vi "DCON Action Engine.vi"(4 "Index\\Channel":i32, 5 "AO Value":dbl, 6 "Action":T4, 7 "DAQDevices":T3[](array[typedef]), 8 "error in (no error)":errorcluster, 9 "DO Value":bool, 10 "Device Name":T1, 11 "IO In":refnum<class "IO.lvclass">) -> (0 "error out":errorcluster, 1 "Status Out":T2, 2 "Channel Data":variant, 3 "IO Out":refnum<class "IO.lvclass">)   [LabVIEW 2022 SP3, in "IO.lvclass"]
uses:
  IO.lvclass
  Typedefs/DCON Action Engine-States.ctl
  Typedefs/DCON_DeviceConfig--Cluster.ctl
  Typedefs/DCON Private Data.ctl
  Typedefs/Device Names.ctl
  <vilib>/Instr/_visa.llb/VISA Flush IO Buffer Mask.ctl
  98b29336-fba3-426d-ab06-4e330d8353b0.vi
  <userlib>/_OpenG.lib/array/array.llb/Remove Duplicates from 1D Array (String)__ogtk.vi
  <userlib>/_OpenG.lib/array/array.llb/Delete Elements from 1D Array (U32)__ogtk.vi
  <vilib>/Instr/_visa.llb/VISA Configure Serial Port (Instr).vi
panel:
  out "read buffer 4":string
  out "read buffer 3":string
  out "read buffer 2":string
  out "read buffer":string
  out "output 1":i32
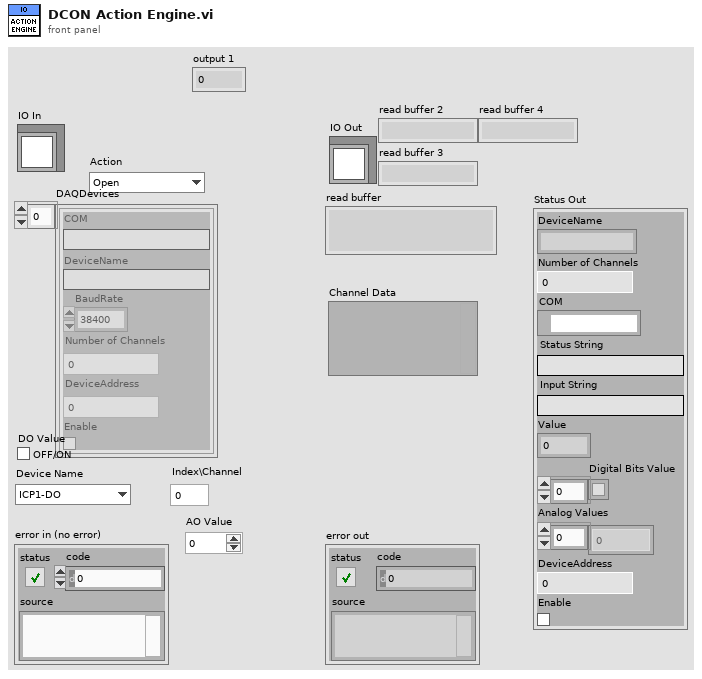
[diagram p1: front panel]
types:
  T1 = typedef "IO.lvclass/Device Names.ctl" = enum16{"ICP1-DO", "ICP2-DI", "ICP2-DO", "ICP1-AI", "ICP1-AO", "ICP2-AO"}
  T2 = typedef "IO.lvclass/DCON Private Data.ctl" = cluster{"DeviceName":string, "Number of Channels":i32, "COM":refnum<visa-resource-name>, "Status String":string, "Input String":string, "Value ":i32, "Digital Bits Value":bool[], "Analog Values":dbl[], "DeviceAddress":i32, "Enable":bool}
  T3 = typedef "IO.lvclass/DCON_DeviceConfig--Cluster.ctl" = cluster{"COM":string, "DeviceName":string, "BaudRate":u32, "Number of Channels":i32, "DeviceAddress":i32, "Enable":bool}
  T4 = typedef "DCON Action Engine-States.ctl" = enum16{"Open", "Close", "Set DO Value", "Get Digital Status", "Get Data", "Get AI Status", "Set AO Value", "Get AO Status"}
  T5 = typedef "VISA Flush IO Buffer Mask.ctl" = u16
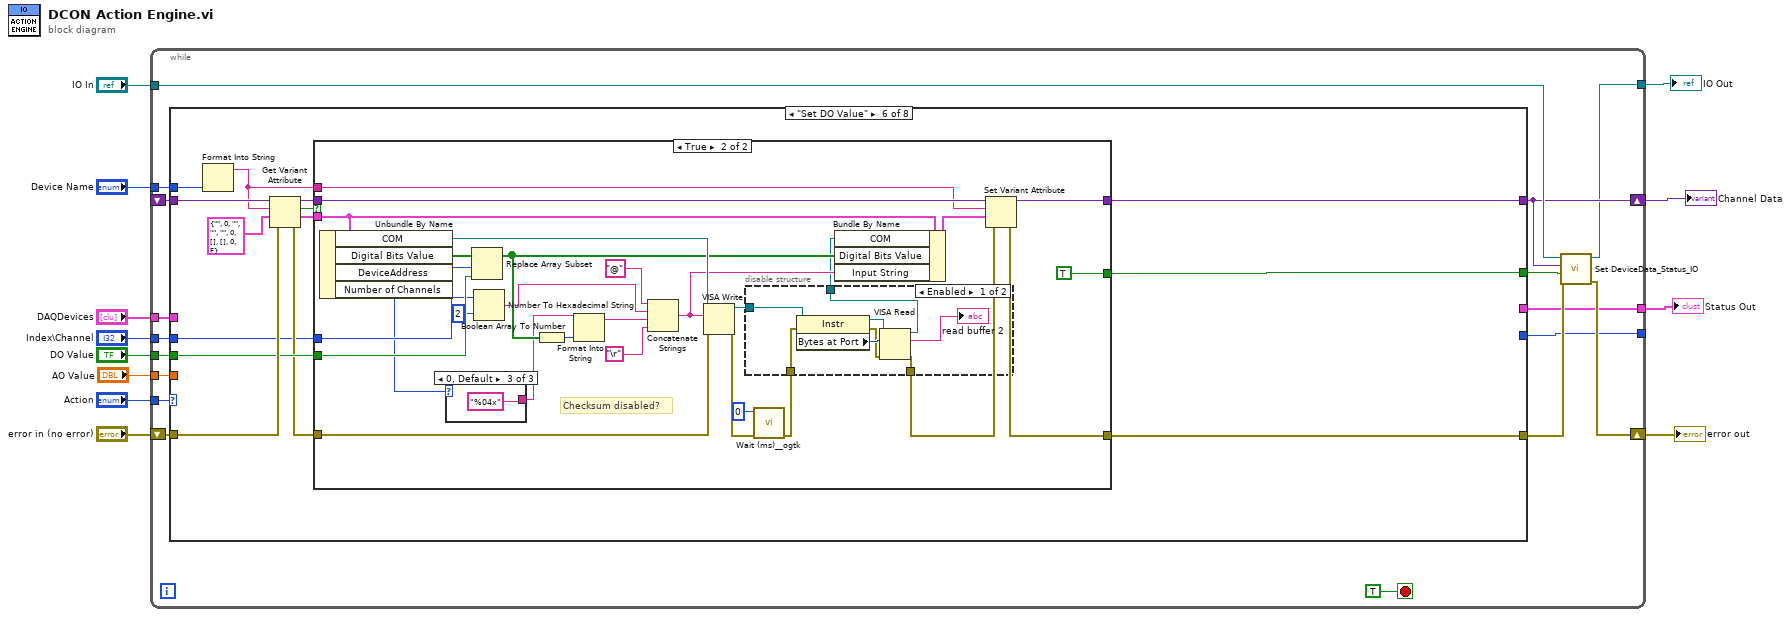
[diagram p0: block diagram]
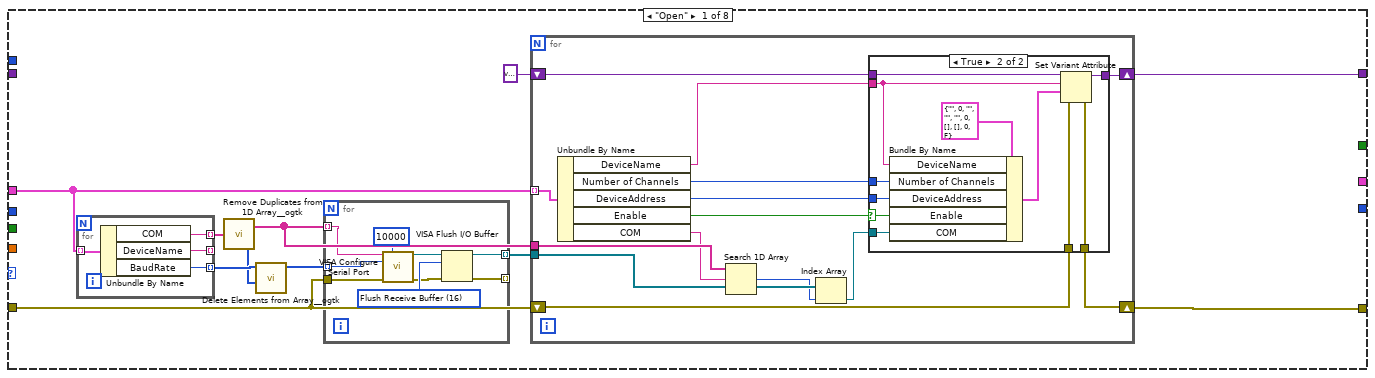
[diagram p2: hidden frame]
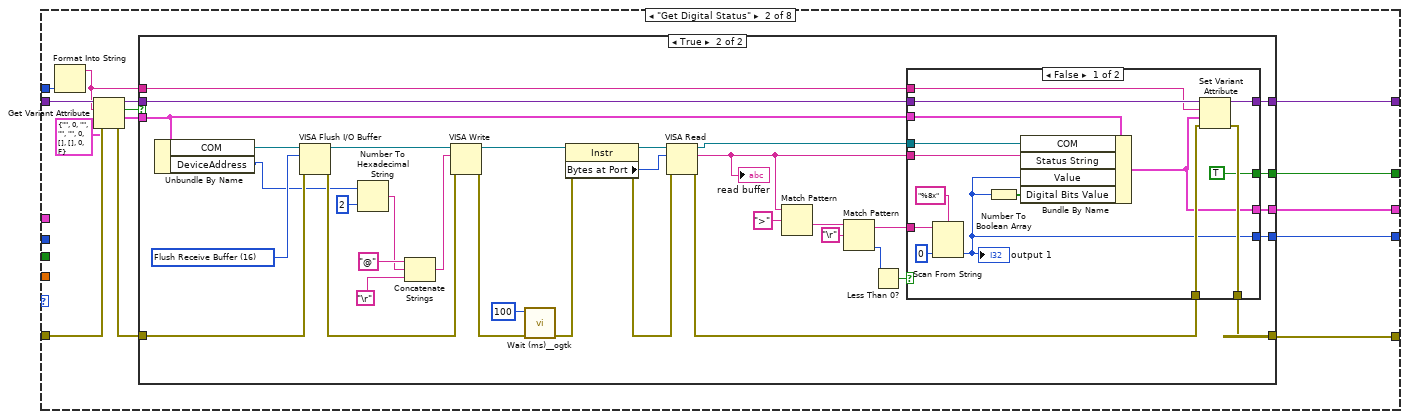
[diagram p4: hidden frame]
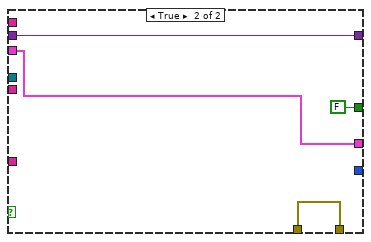
[diagram p6: hidden frame]
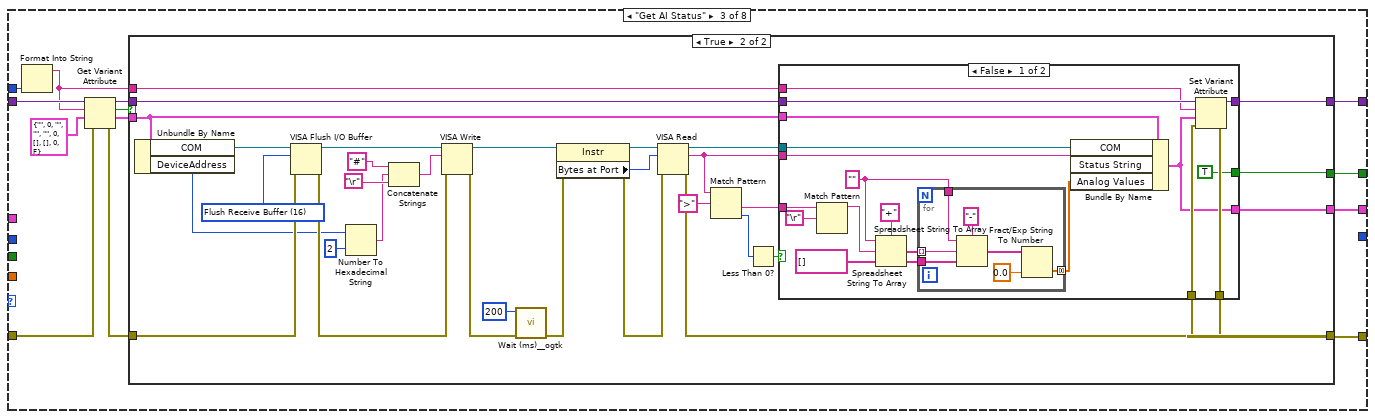
[diagram p7: hidden frame]
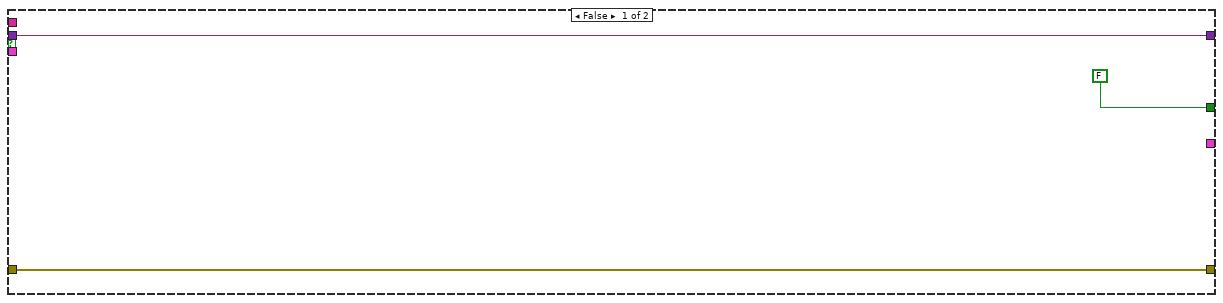
[diagram p8: hidden frame]
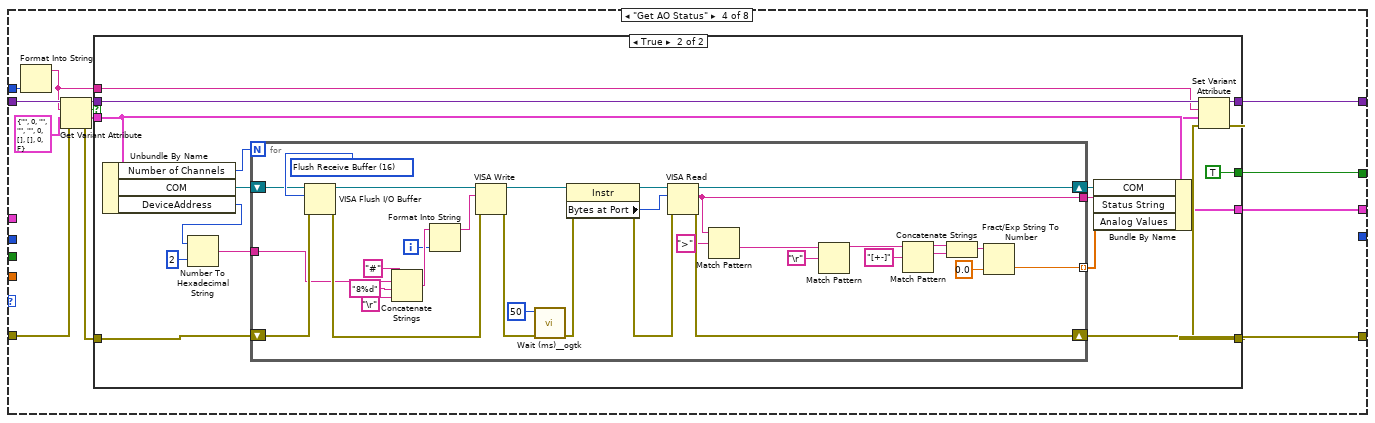
[diagram p10: hidden frame]
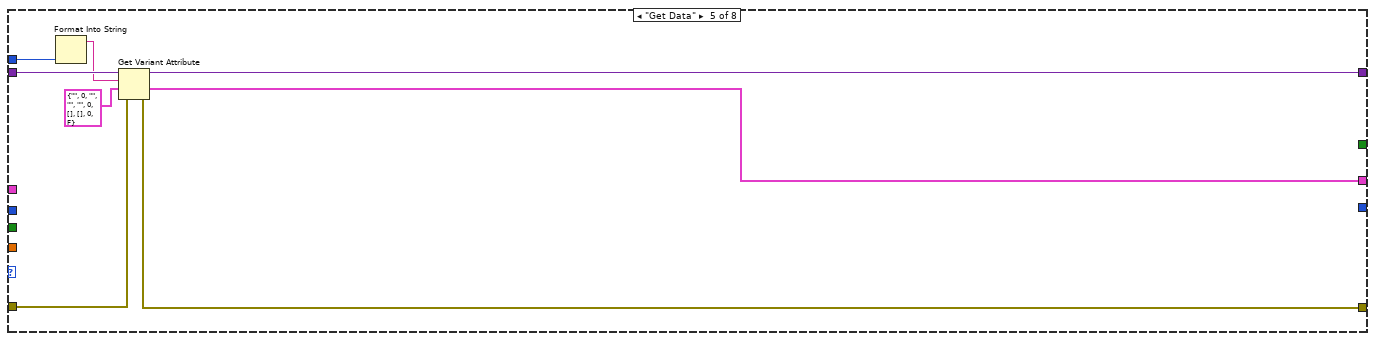
[diagram p12: hidden frame]
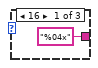
[diagram p14: hidden frame]
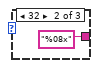
[diagram p15: hidden frame]
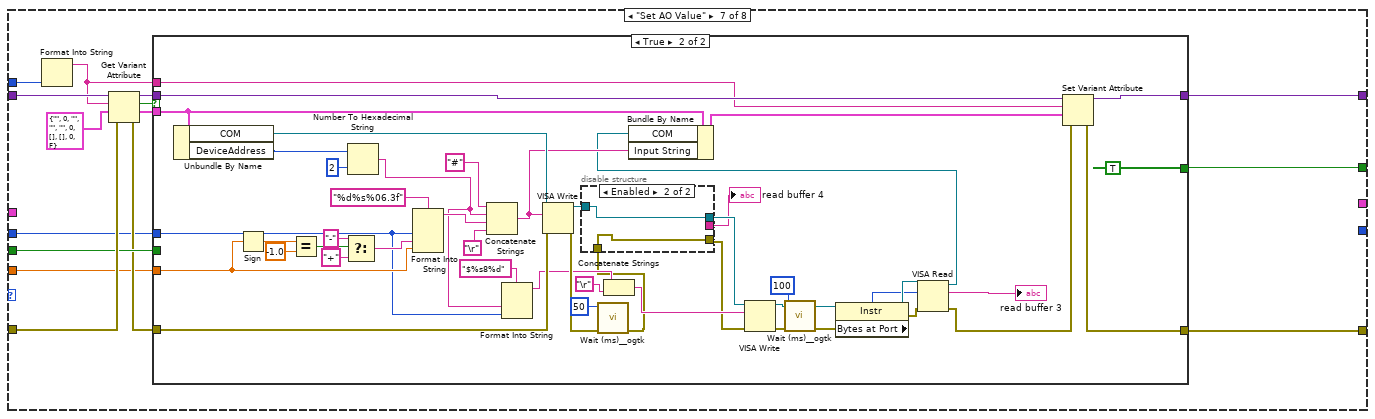
[diagram p17: hidden frame]
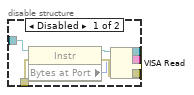
[diagram p19: hidden frame]
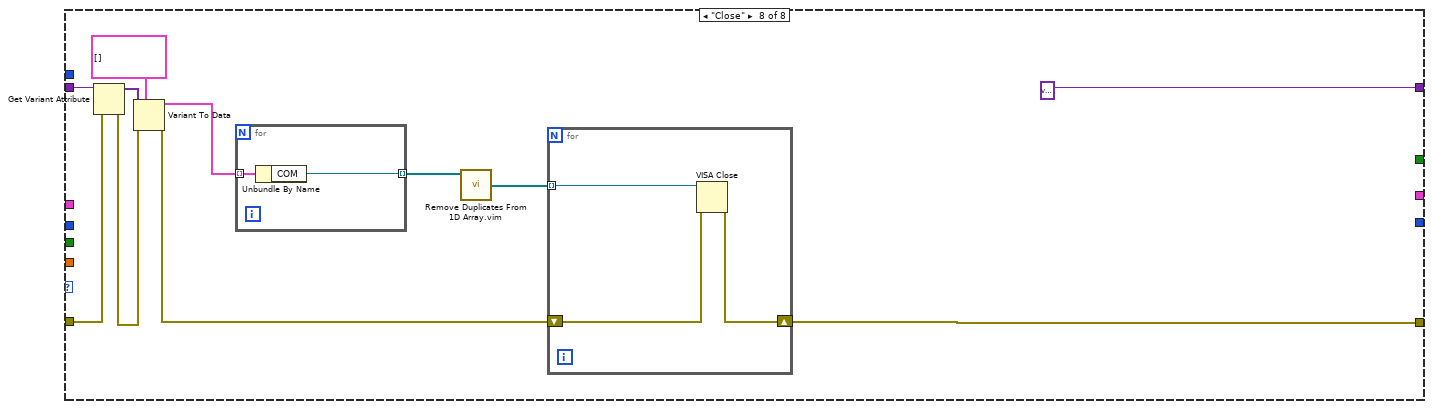
[diagram p20: hidden frame]
diagram:
  n1 = while {
    tunnel: "Action" -> [w28]
    tunnel: "DAQDevices" -> [w27]
    shift-right: [w19] -> w8
    shift-left: "error in (no error)" -> [w26]
    shift-right: [w21] -> w7
    shift-left: _ -> [w25]
    tunnel: "Device Name" -> [w24]
    tunnel: "DO Value" -> [w23]
    tunnel: "IO In" -> [w22]
    tunnel: [w18] -> w5
    tunnel: [w17] -> _
    tunnel: [w16] -> w4
    tunnel: "Index\\Channel" -> [w15]
    tunnel: "AO Value" -> [w14]
    stop <- TRUE stop-if-true
    n2 = case shown="\"Set DO Value\"" w28 {
      tunnel: w27 -> [w37 _ _ _ _ _ _ _]
      tunnel: w26 -> [w30 w92 w161 w237 w297 w311 w370 w435]
      tunnel: [w40 w89 w157 w233 w291 w307 w366 w440] -> w20
      tunnel: [w38 w88 w156 w232 w292 w306 w365 variant] -> w21
      tunnel: w25 -> [_ w94 w163 w239 w298 w312 w371 w439]
      tunnel: w24 -> [_ w85 w153 w229 w295 w302 w361 _]
      tunnel: w23 -> [_ _ _ _ _ w305 w364 _]
      tunnel: [_ w87 _ _ _ _ _ _] -> w17
      tunnel: [_ w86 w154 w230 w293 _ _ _] -> w16
      tunnel: w15 -> [_ _ _ _ _ w300 w359 _]
      tunnel: w14 -> [_ _ _ _ _ _ w358 _]
      tunnel: [_ w83 w151 w227 _ w299 w357 _] -> w13
      frame "Open" {
        n3 = for {
          tunnel: w37 -> [w53] mode=indexing
          tunnel: [w52] -> w36 mode=indexing
          tunnel: [w51] -> _ mode=indexing
          tunnel: [w50] -> w35 mode=indexing
          n4 = Unbundle By Name(w53) -> ("COM"=w52:string, "DeviceName"=w51:string, "BaudRate"=w50:u32)
        }
        n5 = call-poly <userlib>:"Remove Duplicates from 1D Array__ogtk.vi"("Input Array"=w36) -> ("Output Array"=w32:string[], "indices of removed elements"=w34:i32[])
        n6 = call-poly <userlib>:"Delete Elements from Array__ogtk.vi"("indices"=w34, "array"=w35) -> ("array w/ subset deleted"=w33:u32[])  [unwired: 8 in, 1 out]
        n7 = for {
          tunnel: w32 -> [w46] mode=indexing
          tunnel: w33 -> [w45] mode=indexing
          tunnel: [w44] -> w31 mode=indexing
          tunnel: [w43] -> _ mode=indexing
          tunnel: w30 -> [w41]
          w48 = T5 16 items=["Flush Receive Buffer"=16, "Write Transmit Buffer to Device"=32, "Flush Receive Buffer (No I/O)"=64, "Flush Transmit Buffer"=128] ("Mask")
          n8 = call-poly "VISA Configure Serial Port"("VISA resource name"=w46, "timeout (10sec)"=u32 10000, "baud rate (9600)"=w45, "error in (no error)"=w41) -> ("VISA resource name out"=w49:refnum<visa-resource-name>, "error out"=w42:errorcluster)  [unwired: 10 in]
          n9 = VISA Flush I/O Buffer(VISA resource name=w49, mask (16)=w48, error in (no error)=w42) -> (VISA resource name out=w44:refnum<visa-resource-name>, error out=w43:errorcluster)
        }
        n10 = for {
          tunnel: w37 -> [w67] mode=indexing
          shift-right: [w64] -> w40
          shift-left: w30 -> [w57]
          shift-right: [w65] -> w38
          shift-left: variant -> [w66]
          tunnel: w32 -> [w60]
          tunnel: w31 -> [w59]
          n11 = Unbundle By Name(w67) -> ("DeviceName"=w63:string, "Number of Channels"=w62:i32, "DeviceAddress"=w61:i32, "Enable"=w54:bool, "COM"=w56:string)
          n12 = Search 1D Array(1D array=w60, element=w56) -> (index of element=w58:i32)  [unwired: 1 in]
          n13 = Index Array(array=w59, index=w58) -> (element=w55:refnum<visa-resource-name>)
          n14 = case shown="True" w54 {
            selector: w54 -> [_ w70]
            tunnel: w66 -> [w69 w79]
            tunnel: [w69 w77] -> w65
            tunnel: [w68 w76] -> w64
            tunnel: w63 -> [_ w75]
            tunnel: w62 -> [_ w74]
            tunnel: w61 -> [_ w73]
            tunnel: w57 -> [w68 w72]
            tunnel: w55 -> [_ w71]
            frame False {
            }
            frame True {
              n15 = Bundle By Name(cluster=T2 {"DeviceName"="", "Number of Channels"=0, "COM"="", "Status String"="", "Input String"="", "Value "=0, "Digital Bits Value"=[], "Analog Values"=[], "DeviceAddress"=0, "Enable"=FALSE} ("DCON Private Data"), "DeviceName"=w75, "Number of Channels"=w74, "DeviceAddress"=w73, "Enable"=w70, "COM"=w71) -> (w78:T2)
              n16 = Set Variant Attribute(Variant=w79, name=w75, value=w78, error in=w72) -> (Variant out=w77:variant, error out=w76:errorcluster)  [unwired: 1 out]
            }
          }
        }
      }
      frame "Get Digital Status" {
        n17 = Format Into String(w85) -> (resulting string=w84:string)  [unwired: 3 in, 1 out]
        n18 = Get Variant Attribute(Variant=w94, name=w84, default value (empty Variant)=T2 {"DeviceName"="", "Number of Channels"=0, "COM"="", "Status String"="", "Input String"="", "Value "=0, "Digital Bits Value"=[], "Analog Values"=[], "DeviceAddress"=0, "Enable"=FALSE} ("DCON Private Data"), error in=w92) -> (duplicate Variant=w90:variant, found=w81:bool, value=w82:T2, error out=w93:errorcluster)
        n19 = case shown="True" w81 {
          tunnel: w93 -> [w95 w131]
          tunnel: w90 -> [w96 w110]
          tunnel: w84 -> [_ w109]
          tunnel: w82 -> [_ w108]
          tunnel: [w95 w106] -> w89
          tunnel: [w96 w105] -> w88
          tunnel: [_ w103] -> w87
          tunnel: [_ w104] -> w86
          tunnel: [_ w102] -> w83
          frame False {
          }
          frame True {
            w118 = T5 16 items=["Flush Receive Buffer"=16, "Write Transmit Buffer to Device"=32, "Flush Receive Buffer (No I/O)"=64, "Flush Transmit Buffer"=128] ("Mask")
            n20 = Unbundle By Name(w108) -> ("COM"=w111:refnum<visa-resource-name>, "DeviceAddress"=w100:i32)
            n21 = VISA Flush I/O Buffer(VISA resource name=w111, mask (16)=w118, error in (no error)=w131) -> (VISA resource name out=w117:refnum<visa-resource-name>, error out=w116:errorcluster)
            n22 = Number To Hexadecimal String(1:i16 2 ("width (-)"), 2:w100) -> (0:w99:string)
            n23 = Concatenate Strings("@" ("string"), w99, "\r") -> (w127:string)
            n24 = VISA Write(VISA resource name=w117, write buffer=w127, error in (no error)=w116) -> (VISA resource name out=w122:refnum<visa-resource-name>, error out=w121:errorcluster)  [unwired: 1 out]
            n25 = call <userlib>:"Wait (ms)__ogtk.vi"("error in (no error)"=w121, "milliseconds to wait"=u32 100) -> ("error out"=w120:errorcluster)  [unwired: 8 in, 1 out]
            n26 = property class="Instr"(reference=w122, error in=w120) -> (reference out=w125:refnum<visa-resource-name>, error out=w124:errorcluster, "Bytes at Port"=w123:u32)
            n27 = VISA Read(VISA resource name=w125, byte count=w123, error in (no error)=w124) -> (VISA resource name out=w130:refnum<visa-resource-name>, read buffer=w129:string, error out=w107:errorcluster)  [unwired: 1 out]
            "read buffer" <- w129
            n28 = Match Pattern(string=w129, regular expression=">") -> (after substring=w113:string)  [unwired: 1 in, 3 out]
            n29 = Match Pattern(string=w113, regular expression="\r") -> (before substring=w112:string, offset past match=w98:i32)  [unwired: 1 in, 2 out]
            n30 = Less Than 0?(x=w98) -> (x < 0?=w97:bool)
            n31 = case shown="False" w97 {
              tunnel: w130 -> [w146 _]
              tunnel: w129 -> [w145 _]
              tunnel: w112 -> [w144 _]
              tunnel: w110 -> [w142 w148]
              tunnel: w109 -> [w141 _]
              tunnel: w108 -> [w140 w150]
              tunnel: w107 -> [w139 w147]
              tunnel: [w138 w147] -> w106
              tunnel: [w137 w148] -> w105
              tunnel: [w135 w150] -> w104
              tunnel: [w134 _] -> w103
              tunnel: [TRUE FALSE] -> w102
              frame False {
                n32 = Scan From String(format string="%8x", input string=w144, default 1=0) -> (output 1=w134:i32)  [unwired: 2 in, 3 out]
                "output 1" <- w134
                n33 = Number To Boolean Array(number=w134) -> (Boolean array=w133:bool[])
                n34 = Bundle By Name(cluster=w140, "COM"=w146, "Status String"=w145, "Value"=w134, "Digital Bits Value"=w133) -> (w135:T2)
                n35 = Set Variant Attribute(Variant=w142, name=w141, value=w135, error in=w139) -> (Variant out=w137:variant, error out=w138:errorcluster)  [unwired: 1 out]
              }
              frame True {
              }
            }
          }
        }
      }
      frame "Get AI Status" {
        n36 = Format Into String(w153) -> (resulting string=w152:string)  [unwired: 3 in, 1 out]
        n37 = Get Variant Attribute(Variant=w163, name=w152, default value (empty Variant)=T2 {"DeviceName"="", "Number of Channels"=0, "COM"="", "Status String"="", "Input String"="", "Value "=0, "Digital Bits Value"=[], "Analog Values"=[], "DeviceAddress"=0, "Enable"=FALSE} ("DCON Private Data"), error in=w161) -> (duplicate Variant=w159:variant, found=w155:bool, value=w158:T2, error out=w162:errorcluster)
        n38 = case shown="True" w155 {
          tunnel: w162 -> [w165 w198]
          tunnel: w159 -> [w166 w182]
          tunnel: w152 -> [_ w181]
          tunnel: w158 -> [_ w180]
          tunnel: [w165 w178] -> w157
          tunnel: [w166 w177] -> w156
          tunnel: [_ w176] -> w154
          tunnel: [FALSE w167] -> w151
          frame False {
          }
          frame True {
            w186 = T5 16 items=["Flush Receive Buffer"=16, "Write Transmit Buffer to Device"=32, "Flush Receive Buffer (No I/O)"=64, "Flush Transmit Buffer"=128] ("Mask")
            n39 = Unbundle By Name(w180) -> ("COM"=w183:refnum<visa-resource-name>, "DeviceAddress"=w171:i32)
            n40 = VISA Flush I/O Buffer(VISA resource name=w183, mask (16)=w186, error in (no error)=w198) -> (VISA resource name out=w185:refnum<visa-resource-name>, error out=w184:errorcluster)
            n41 = Number To Hexadecimal String(1:i16 2 ("width (-)"), 2:w171) -> (0:w170:string)
            n42 = Concatenate Strings("#" ("string"), w170, "\r") -> (w195:string)
            n43 = VISA Write(VISA resource name=w185, write buffer=w195, error in (no error)=w184) -> (VISA resource name out=w190:refnum<visa-resource-name>, error out=w189:errorcluster)  [unwired: 1 out]
            n44 = call <userlib>:"Wait (ms)__ogtk.vi"("error in (no error)"=w189, "milliseconds to wait"=u32 200) -> ("error out"=w188:errorcluster)  [unwired: 8 in, 1 out]
            n45 = property class="Instr"(reference=w190, error in=w188) -> (reference out=w193:refnum<visa-resource-name>, error out=w192:errorcluster, "Bytes at Port"=w191:u32)
            n46 = VISA Read(VISA resource name=w193, byte count=w191, error in (no error)=w192) -> (VISA resource name out=w197:refnum<visa-resource-name>, read buffer=w173:string, error out=w179:errorcluster)  [unwired: 1 out]
            n47 = Match Pattern(string=w173, regular expression=">") -> (after substring=w174:string, offset past match=w169:i32)  [unwired: 1 in, 2 out]
            n48 = Less Than 0?(x=w169) -> (x < 0?=w168:bool)
            n49 = case shown="False" w168 {
              tunnel: w197 -> [w216 _]
              tunnel: w182 -> [w215 w226]
              tunnel: w181 -> [w214 _]
              tunnel: w180 -> [w213 w225]
              tunnel: w179 -> [w212 w224]
              tunnel: [w211 w224] -> w178
              tunnel: [w210 w226] -> w177
              tunnel: [w209 w225] -> w176
              tunnel: w174 -> [w207 _]
              tunnel: w173 -> [w200 _]
              tunnel: [TRUE _] -> w167
              frame False {
                w203 = string[] []
                w202 = "" ("format string")
                n50 = Match Pattern(string=w207, regular expression="\r") -> (before substring=w206:string)  [unwired: 1 in, 3 out]
                n51 = Spreadsheet String To Array(delimiter (Tab)="+", format string=w202, spreadsheet string=w206, array type (2D Dbl)=w203) -> (array=w204:string[])
                n52 = for {
                  tunnel: w204 -> [w222] mode=indexing
                  tunnel: [w219] -> w201 mode=concatenating
                  tunnel: w203 -> [w218]
                  tunnel: w202 -> [w217]
                  n53 = Spreadsheet String To Array(delimiter (Tab)="-", format string=w217, spreadsheet string=w222, array type (2D Dbl)=w218) -> (array=w221:string[])
                  n54 = Fract/Exp String To Number(string=w221, default (0 dbl)=0.0) -> (number=w219:dbl[])  [unwired: 2 in, 1 out]
                }
                n55 = Bundle By Name(cluster=w213, "COM"=w216, "Status String"=w200, "Analog Values"=w201) -> (w209:T2)
                n56 = Set Variant Attribute(Variant=w215, name=w214, value=w209, error in=w212) -> (Variant out=w210:variant, error out=w211:errorcluster)  [unwired: 1 out]
              }
              frame True {
              }
            }
          }
        }
      }
      frame "Get AO Status" {
        n57 = Format Into String(w229) -> (resulting string=w228:string)  [unwired: 3 in, 1 out]
        n58 = Get Variant Attribute(Variant=w239, name=w228, default value (empty Variant)=T2 {"DeviceName"="", "Number of Channels"=0, "COM"="", "Status String"="", "Input String"="", "Value "=0, "Digital Bits Value"=[], "Analog Values"=[], "DeviceAddress"=0, "Enable"=FALSE} ("DCON Private Data"), error in=w237) -> (duplicate Variant=w235:variant, found=w231:bool, value=w234:T2, error out=w238:errorcluster)
        n59 = case shown="True" w231 {
          tunnel: w238 -> [w240 w258]
          tunnel: w235 -> [w241 w255]
          tunnel: w228 -> [_ w254]
          tunnel: w234 -> [_ w253]
          tunnel: [w240 w251] -> w233
          tunnel: [w241 w250] -> w232
          tunnel: [_ w249] -> w230
          tunnel: [_ TRUE] -> w227
          frame False {
          }
          frame True {
            n60 = Unbundle By Name(w253) -> ("Number of Channels"=w246:i32, "COM"=w256:refnum<visa-resource-name>, "DeviceAddress"=w243:i32)
            n61 = Number To Hexadecimal String(1:i16 2 ("width (-)"), 2:w243) -> (0:w242:string)
            n62 = for {
              N: w246 -> [_]
              tunnel: [w272] -> w248 mode=indexing
              tunnel: [w271] -> w247
              shift-right: [w276] -> w252
              shift-left: w258 -> [w290]
              shift-right: [w289] -> w257
              shift-left: w256 -> [w277]
              tunnel: w242 -> [w259]
              i -> [w263]
              w280 = T5 16 items=["Flush Receive Buffer"=16, "Write Transmit Buffer to Device"=32, "Flush Receive Buffer (No I/O)"=64, "Flush Transmit Buffer"=128] ("Mask")
              n63 = VISA Flush I/O Buffer(VISA resource name=w277, mask (16)=w280, error in (no error)=w290) -> (VISA resource name out=w279:refnum<visa-resource-name>, error out=w278:errorcluster)
              n64 = Concatenate Strings("#" ("string"), w259, "8%d" ("string"), "\r") -> (w264:string)
              n65 = Format Into String(format string=w264, w263) -> (resulting string=w262:string)  [unwired: 2 in, 1 out]
              n66 = VISA Write(VISA resource name=w279, write buffer=w262, error in (no error)=w278) -> (VISA resource name out=w284:refnum<visa-resource-name>, error out=w283:errorcluster)  [unwired: 1 out]
              n67 = call <userlib>:"Wait (ms)__ogtk.vi"("error in (no error)"=w283, "milliseconds to wait"=u32 50) -> ("error out"=w282:errorcluster)  [unwired: 8 in, 1 out]
              n68 = property class="Instr"(reference=w284, error in=w282) -> (reference out=w287:refnum<visa-resource-name>, error out=w286:errorcluster, "Bytes at Port"=w285:u32)
              n69 = VISA Read(VISA resource name=w287, byte count=w285, error in (no error)=w286) -> (VISA resource name out=w289:refnum<visa-resource-name>, read buffer=w271:string, error out=w276:errorcluster)  [unwired: 1 out]
              n70 = Match Pattern(string=w271, regular expression=">") -> (after substring=w273:string)  [unwired: 1 in, 3 out]
              n71 = Match Pattern(string=w273, regular expression="\r") -> (before substring=w269:string)  [unwired: 1 in, 3 out]
              n72 = Match Pattern(string=w269, regular expression="[+-]") -> (before substring=w267:string, match substring=w266:string)  [unwired: 1 in, 2 out]
              n73 = Concatenate Strings(w267, w266) -> (w265:string)
              n74 = Fract/Exp String To Number(string=w265, default (0 dbl)=0.0) -> (number=w272:dbl)  [unwired: 2 in, 1 out]
            }
            n75 = Bundle By Name(cluster=w253, "COM"=w257, "Status String"=w247, "Analog Values"=w248) -> (w249:T2)
            n76 = Set Variant Attribute(Variant=w255, name=w254, value=w249, error in=w252) -> (Variant out=w250:variant, error out=w251:errorcluster)  [unwired: 1 out]
          }
        }
      }
      frame "Get Data" {
        n77 = Format Into String(w295) -> (resulting string=w294:string)  [unwired: 3 in, 1 out]
        n78 = Get Variant Attribute(Variant=w298, name=w294, default value (empty Variant)=T2 {"DeviceName"="", "Number of Channels"=0, "COM"="", "Status String"="", "Input String"="", "Value "=0, "Digital Bits Value"=[], "Analog Values"=[], "DeviceAddress"=0, "Enable"=FALSE} ("DCON Private Data"), error in=w297) -> (duplicate Variant=w292:variant, value=w293:T2, error out=w291:errorcluster)  [unwired: 1 out]
      }
      frame "Set DO Value" {
        n79 = Format Into String(w302) -> (resulting string=w301:string)  [unwired: 3 in, 1 out]
        n80 = Get Variant Attribute(Variant=w312, name=w301, default value (empty Variant)=T2 {"DeviceName"="", "Number of Channels"=0, "COM"="", "Status String"="", "Input String"="", "Value "=0, "Digital Bits Value"=[], "Analog Values"=[], "DeviceAddress"=0, "Enable"=FALSE} ("DCON Private Data"), error in=w311) -> (duplicate Variant=w309:variant, found=w303:bool, value=w308:T2, error out=w304:errorcluster)
        n81 = case shown="True" w303 {
          tunnel: w309 -> [w314 w343]
          tunnel: w301 -> [_ w342]
          tunnel: w308 -> [_ w341]
          tunnel: [w313 w339] -> w307
          tunnel: [w314 w338] -> w306
          tunnel: w305 -> [_ w329]
          tunnel: w304 -> [w313 w333]
          tunnel: w300 -> [_ w327]
          tunnel: [_ TRUE] -> w299
          frame False {
          }
          frame True {
            # "Checksum disabled?"
            n82 = Unbundle By Name(w341) -> ("COM"=w337:refnum<visa-resource-name>, "Digital Bits Value"=w330:bool[], "DeviceAddress"=w323:i32, "Number of Channels"=w316:i32)
            n83 = case shown="0, Default" w316 {
              tunnel: ["%04x" ("format string") "%08x" ("format string") "%04x" ("format string")] -> w315
              frame 16 {
              }
              frame 32 {
              }
              frame 0, Default {
              }
            }
            n84 = Replace Array Subset(array=w330, new element=w329, index=w327) -> (w326:bool[])
            n85 = Number To Hexadecimal String(1:i16 2 ("width (-)"), 2:w323) -> (0:w322:string)
            n86 = Boolean Array To Number(Boolean array=w326) -> (number=w328:u32)
            n87 = Format Into String(format string=w315, w328) -> (resulting string=w335:string)  [unwired: 2 in, 1 out]
            n88 = Concatenate Strings("@" ("string"), w322, w335, "\r") -> (w331:string)
            n89 = VISA Write(VISA resource name=w337, write buffer=w331, error in (no error)=w333) -> (VISA resource name out=w318:refnum<visa-resource-name>, error out=w332:errorcluster)  [unwired: 1 out]
            n90 = call <userlib>:"Wait (ms)__ogtk.vi"("error in (no error)"=w332, "milliseconds to wait"=u32 0) -> ("error out"=w320:errorcluster)  [unwired: 8 in, 1 out]
            n91 = disable-structure shown="Enabled" {
              disable-tunnel: w320 -> [w348 w356]
              disable-tunnel: [w354 w356] -> w319
              disable-tunnel: w318 -> [w351 w355]
              disable-tunnel: [w350 w355] -> w317
              frame Enabled {
                n92 = property class="Instr"(reference=w351, error in=w348) -> (reference out=w352:refnum<visa-resource-name>, error out=w347:errorcluster, "Bytes at Port"=w349:u32)
                n93 = VISA Read(VISA resource name=w352, byte count=w349, error in (no error)=w347) -> (VISA resource name out=w350:refnum<visa-resource-name>, read buffer=→"read buffer 2":string, error out=w354:errorcluster)  [unwired: 1 out]
              }
              frame Disabled {
              }
            }
            n94 = Bundle By Name(cluster=w341, "COM"=w317, "Digital Bits Value"=w326, "Input String"=w331) -> (w340:T2)
            n95 = Set Variant Attribute(Variant=w343, name=w342, value=w340, error in=w319) -> (Variant out=w338:variant, error out=w339:errorcluster)  [unwired: 1 out]
          }
        }
      }
      frame "Set AO Value" {
        n96 = Format Into String(w361) -> (resulting string=w360:string)  [unwired: 3 in, 1 out]
        n97 = Get Variant Attribute(Variant=w371, name=w360, default value (empty Variant)=T2 {"DeviceName"="", "Number of Channels"=0, "COM"="", "Status String"="", "Input String"="", "Value "=0, "Digital Bits Value"=[], "Analog Values"=[], "DeviceAddress"=0, "Enable"=FALSE} ("DCON Private Data"), error in=w370) -> (duplicate Variant=w368:variant, found=w362:bool, value=w367:T2, error out=w363:errorcluster)
        n98 = case shown="True" w362 {
          tunnel: w368 -> [w373 w419]
          tunnel: w360 -> [_ w418]
          tunnel: w367 -> [_ w417]
          tunnel: [w372 w415] -> w366
          tunnel: [w373 w414] -> w365
          tunnel: w364 -> [_ _]
          tunnel: w363 -> [w372 w409]
          tunnel: w359 -> [_ w381]
          tunnel: w358 -> [_ w400]
          tunnel: [_ TRUE] -> w357
          frame False {
          }
          frame True {
            n99 = Unbundle By Name(w417) -> ("COM"=w413:refnum<visa-resource-name>, "DeviceAddress"=w397:i32)
            n100 = Sign(1:w400) -> (0:w405:dbl)
            n101 = Equal?(x=w405, y=-1.0) -> (x = y?=w406:bool)
            n102 = Select(t="-", s=w406, f="+") -> (s? t:f=w401:string)
            n103 = Number To Hexadecimal String(1:i16 2 ("width (-)"), 2:w397) -> (0:w382:string)
            n104 = Format Into String(format string="%d%s%06.3f", w381, w401, w400) -> (resulting string=w396:string)  [unwired: 2 in, 1 out]
            n105 = Concatenate Strings("#" ("string"), w382, w396, "\r") -> (w407:string)
            n106 = Format Into String(format string="$%s8%d" ("write buffer"), w382, w381) -> (resulting string=w380:string)  [unwired: 2 in, 1 out]
            n107 = VISA Write(VISA resource name=w413, write buffer=w407, error in (no error)=w409) -> (VISA resource name out=w376:refnum<visa-resource-name>, error out=w408:errorcluster)  [unwired: 1 out]
            n108 = call <userlib>:"Wait (ms)__ogtk.vi"("error in (no error)"=w408, "milliseconds to wait"=u32 50) -> ("error out"=w378:errorcluster)  [unwired: 8 in, 1 out]
            n109 = disable-structure shown="Enabled" {
              disable-tunnel: w378 -> [w425 w428]
              disable-tunnel: [w424 w428] -> w377
              disable-tunnel: w376 -> [w423 w429]
              disable-tunnel: [w422 w429] -> w375
              disable-tunnel: [w420 _] -> w374
              frame Disabled {
                n110 = property class="Instr"(reference=w423, error in=w425) -> (reference out=w426:refnum<visa-resource-name>, error out=w427:errorcluster, "Bytes at Port"=w421:u32)
                n111 = VISA Read(VISA resource name=w426, byte count=w421, error in (no error)=w427) -> (VISA resource name out=w422:refnum<visa-resource-name>, read buffer=w420:string, error out=w424:errorcluster)  [unwired: 1 out]
              }
              frame Enabled {
              }
            }
            "read buffer 4" <- w374
            n112 = Concatenate Strings(w380, "\r") -> (w394:string)
            n113 = VISA Write(VISA resource name=w375, write buffer=w394, error in (no error)=w377) -> (VISA resource name out=w389:refnum<visa-resource-name>, error out=w391:errorcluster)  [unwired: 1 out]
            n114 = call <userlib>:"Wait (ms)__ogtk.vi"("error in (no error)"=w391, "milliseconds to wait"=u32 100) -> ("error out"=w385:errorcluster)  [unwired: 8 in, 1 out]
            n115 = property class="Instr"(reference=w389, error in=w385) -> (reference out=w387:refnum<visa-resource-name>, error out=w384:errorcluster, "Bytes at Port"=w386:u32)
            n116 = VISA Read(VISA resource name=w387, byte count=w386, error in (no error)=w384) -> (VISA resource name out=w379:refnum<visa-resource-name>, read buffer=→"read buffer 3":string, error out=w390:errorcluster)  [unwired: 1 out]
            n117 = Bundle By Name(cluster=w417, "COM"=w379, "Input String"=w407) -> (w416:T2)
            n118 = Set Variant Attribute(Variant=w419, name=w418, value=w416, error in=w390) -> (Variant out=w414:variant, error out=w415:errorcluster)  [unwired: 1 out]
          }
        }
      }
      frame "Close" {
        n119 = Get Variant Attribute(Variant=w439, error in=w435) -> (values=w438:variant[], error out=w437:errorcluster)  [unwired: 2 in, 2 out]
        n120 = Variant To Data(error in=w437, type=T2[] [], Variant=w438) -> (data=w432:T2[], error out=w436:errorcluster)
        n121 = for {
          tunnel: w432 -> [w442] mode=indexing
          tunnel: [w441] -> w431 mode=indexing
          n122 = Unbundle By Name(w442) -> ("COM"=w441:refnum<visa-resource-name>)
        }
        n123 = call "Remove Duplicates From 1D Array.vim"("array"=w431) -> ("array with duplicates removed"=w430:refnum<visa-resource-name>[])  [unwired: 10 in]
        n124 = for {
          shift-right: [w444] -> w440
          shift-left: w436 -> [w445]
          tunnel: w430 -> [w443] mode=indexing
          n125 = VISA Close(VISA resource name=w443, error in (no error)=w445) -> (error out=w444:errorcluster)
        }
      }
    }
    n126 = call-dynamic "Set DeviceData_Status_IO.vi"("error in (no error)"=w20, "Trigger Event?"=w13, "Device Data"=w21, "IO in"=w22) -> ("error out"=w19:errorcluster, "IO out"=w18:refnum<class "IO.lvclass">)  [unwired: 6 in]
  }
  "error out" <- w8
  "Channel Data" <- w7
  "IO Out" <- w5
  "Status Out" <- w4
